vi "this.move.vi"(5 "main-national data in":T2, 7 "path array":T4[](array[typedef]), 8 "error in (no error)":errorcluster, 9 "Position in":T1, 10 "recy?":bool, 11 "enable":bool) -> (0 "error out":errorcluster, 1 "Position out":T1, 3 "main-national data out":T2, 4 "Position out 2":T1)   [LabVIEW 2019]
uses:
  ctl/path name.ctl
  subVI/move/position cluster.ctl
  ctl/main data-national.ctl
  ctl/position set.ctl
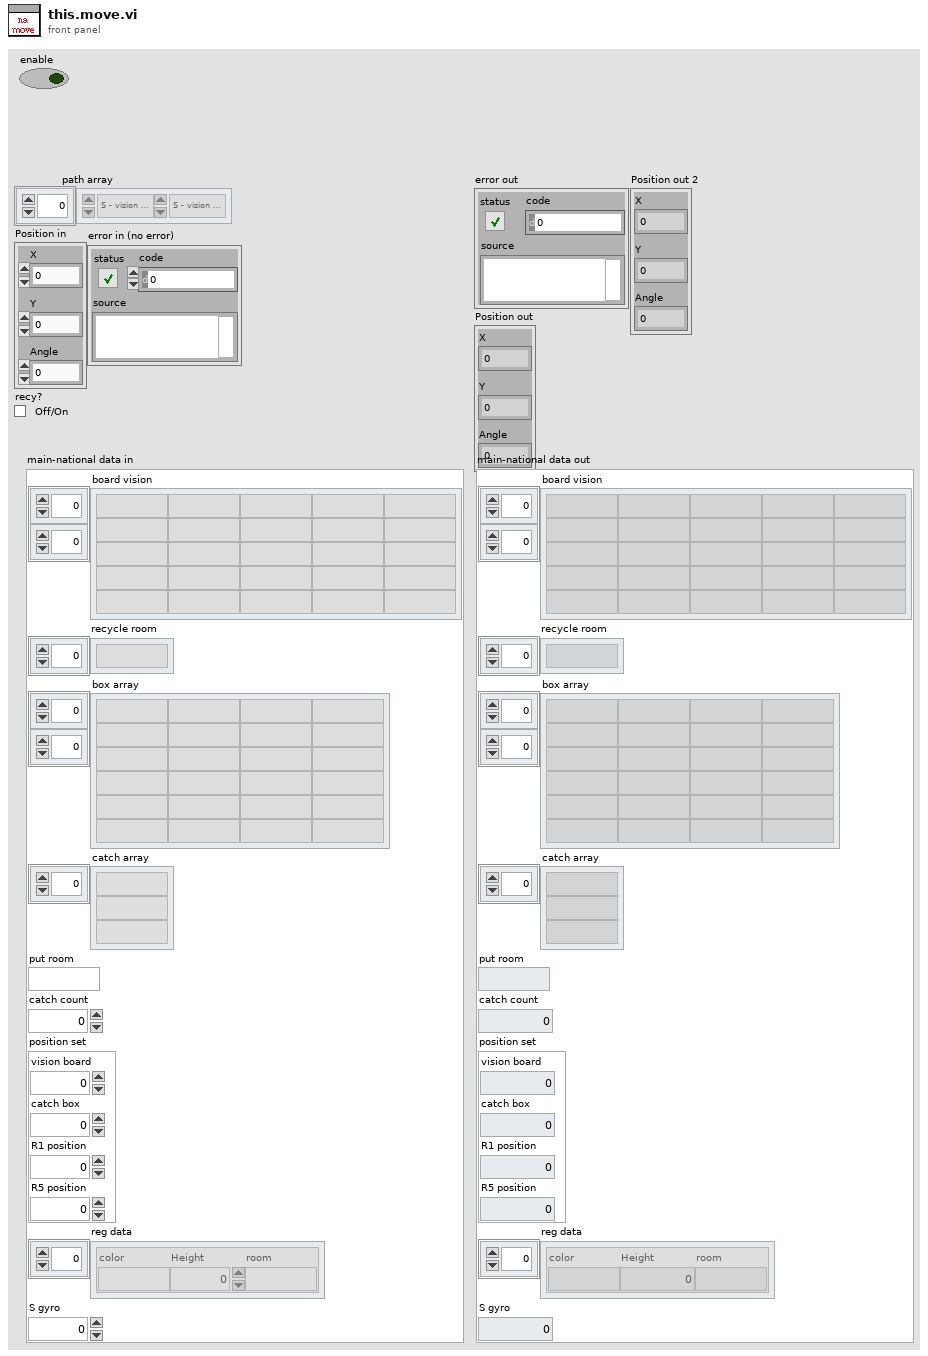
[diagram p1: front panel]
types:
  T1 = typedef "position cluster.ctl" = cluster{"X":dbl, "Y":dbl, "Angle":dbl}
  T2 = typedef "main data-national.ctl" = cluster{"board vision":string[][], "recycle room":string[], "box array":string[][], "catch array":string[], "put room":string, "catch count":dbl, "position set":T3, "reg data":cluster{"color":string, "Height":i32, "room":string}[], "S gyro":dbl}
  T3 = typedef "position set.ctl" = cluster{"vision board":dbl, "catch box":dbl, "R1 position":dbl, "R5 position":dbl}
  T4 = typedef "path name.ctl" = enum16{"S - vision board", "vision board - s out", "s out - room center", "room center - R1", "room center - R2", "room center - R3", "room center - R4", "room center - R5", "R1 - room center", "R2 - room center", "R3 - room center", "R4 - room center", "R5 - room center", "room center - S out", "S-out - recycle", "recycle - S-out", "S-out - s", "s - s-out", "board - box", "box - board", "S out - board", "R1 - R1 d", "R5d - R5", "R3.4-R3", "R3 - R3.2", "- align", "- align.5", "R2 - R2.d", "center align"}
  T5 = typedef "path ctl.ctl" = cluster{"position":T6, "deg":dbl, "en.deg":bool}
  T6 = typedef "position name.ctl" = enum16{"S-zone", "out S", "vision board-vision", "out box", "box catch", "room center", "room right", "room left", "R2", "R4", "only rotate", "out recy", "recycle", "R3", "near board", "box poxition", "R1", "R5", "R1-d", "R5-d", "R3.4", "align center.1", "align center.5", "R2-d", "R2-r", "far center"}
  T7 = typedef "move cluster(VAJ).ctl" = cluster{"X":dbl, "Y":dbl, "degree":dbl, "other":string}
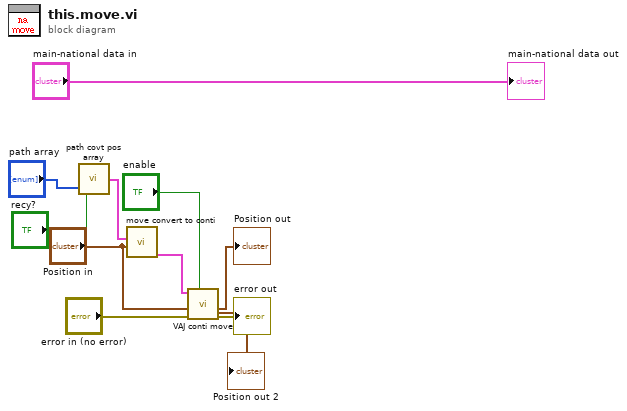
[diagram p0: block diagram]
diagram:
  n1 = call "path covt pos array.vi"("path array"="path array", "recy?"="recy?") -> ("position array"=w10:T5[])
  n2 = call "move convert to conti.vi"("Position"="Position in", "path array"=w10) -> ("VAJ path"=w3:T7[])  [unwired: 8 in, 1 out]
  n3 = call "VAJ conti move.vi"("move?"="enable", "error in (no error)"="error in (no error)", "Position in"="Position in", "move in"=w3) -> ("error out"=→"error out":errorcluster, "Position out"=→"Position out":T1, "Position out 2"=→"Position out 2":T1)  [unwired: 5 in]
  "main-national data out" <- "main-national data in"
